vi "Update Window Surface.vi"(8 "error in":errorcluster, 11 "Window Pointer":u32 format="%.0x") -> (0 "error out":errorcluster)   [LabVIEW 2014, in "LibSDL2.lvlib"]
uses:
  LibSDL2.lvlib
  DLL/SDL2.dll
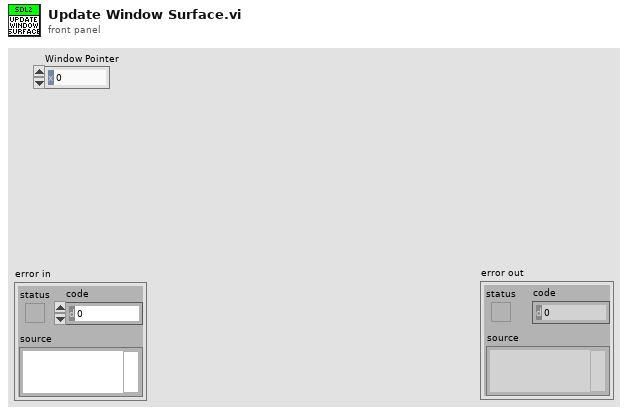
[diagram p1: front panel]
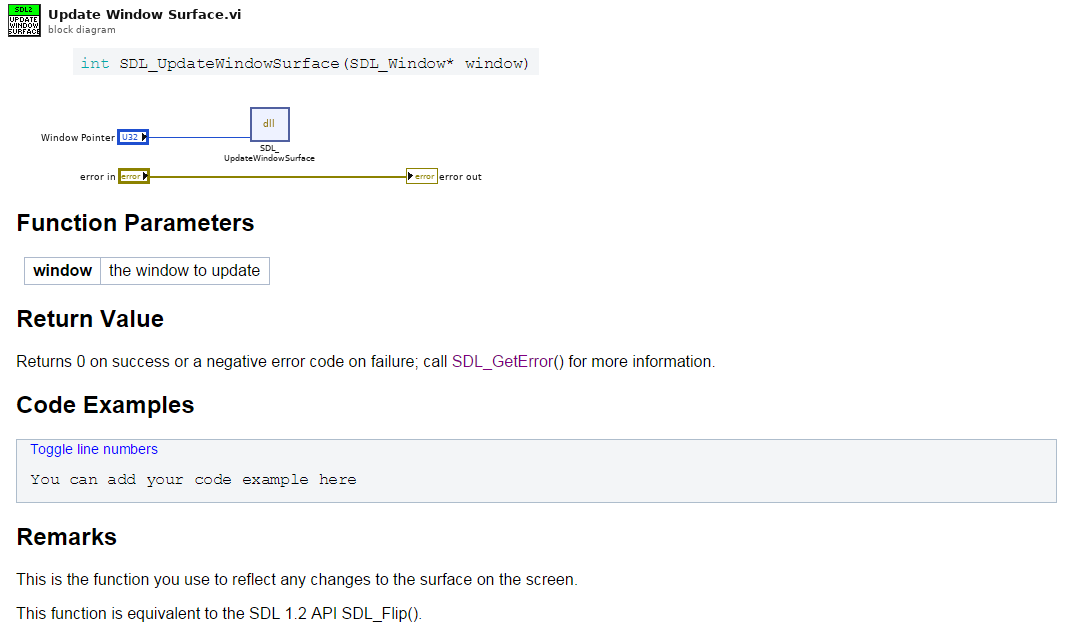
[diagram p0: block diagram]
diagram:
  n1 = dll-call lib="C:/dev/PGS/LabSDL2/Source/LibSDL2 Wrapper/DLL/SDL2.dll" fn="SDL_UpdateWindowSurface"("window"="Window Pointer") -> ()  [unwired: 5 in, 2 out]
  "error out" <- "error in"
